vi "FG COP RBT ServiceSeq.vi"(1 "FG Action (Read)":T2, 2 "RBT ServiceSeq in":T1[](array[typedef])) -> (0 "RBT ServiceSeq out":T1[](array[typedef]))   [LabVIEW 2009]
uses:
  cRIO/Functional Global Variables/Actions for FG's.ctl
  Support Files/ServiceRec.ctl
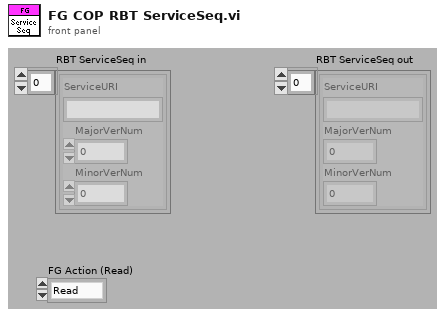
[diagram p1: front panel]
types:
  T1 = typedef "ServiceRec.ctl" = cluster{"ServiceURI":string, "MajorVerNum":u8, "MinorVerNum":u8}
  T2 = typedef "Actions for FG's.ctl" = enum16{"Read", "Write"}
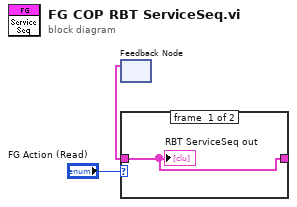
[diagram p0: block diagram]
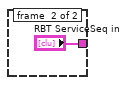
[diagram p2: hidden frame]
diagram:
  n1 = feedback #1() -> (w1:T1[])  [unwired: 1 in]
  n2 = case shown="\"Write\"" "FG Action (Read)" {
    tunnel: w1 -> [w4 _]
    tunnel: [w4 "RBT ServiceSeq in"] -> w2
    frame #0 {
      "RBT ServiceSeq out" <- w4
    }
    frame #1 {
    }
  }
